vi "From Binary.vi"(8 "error in (no error)":errorcluster, 9 "byte order":T1(ring), 10 "Binary":string, 11 "Double Float in":refnum<class "AbsFunc_One Term_DBL.lvclass">) -> (0 "error out":errorcluster, 2 "Remaning Binary":string, 3 "Double Float out":refnum<class "AbsFunc_One Term_DBL.lvclass">)   [LabVIEW 2021, in "AbsFunc_One Term_DBL.lvclass"]
uses:
  AbsFunc_One Term_DBL.lvclass
  AbsFunc_One Term_DBL.lvclass/AbsFunc_One Term_DBL.ctl
  Abs_Types/Double Float/Abs_Double Float.lvclass
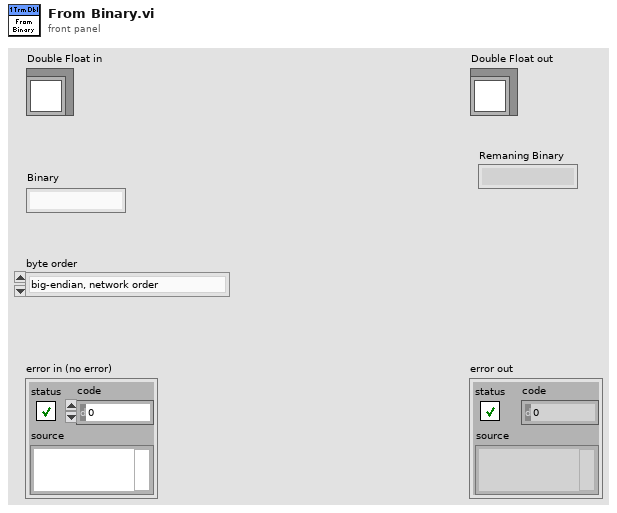
[diagram p1: front panel]
types:
  T1 = enum16{"big-endian, network order", "native, host order", "little-endian"}
  T2 = typedef "One Term_DBL.lvclass/Abstract Type.ctl" = refnum<class "Abs_Double Float.lvclass">
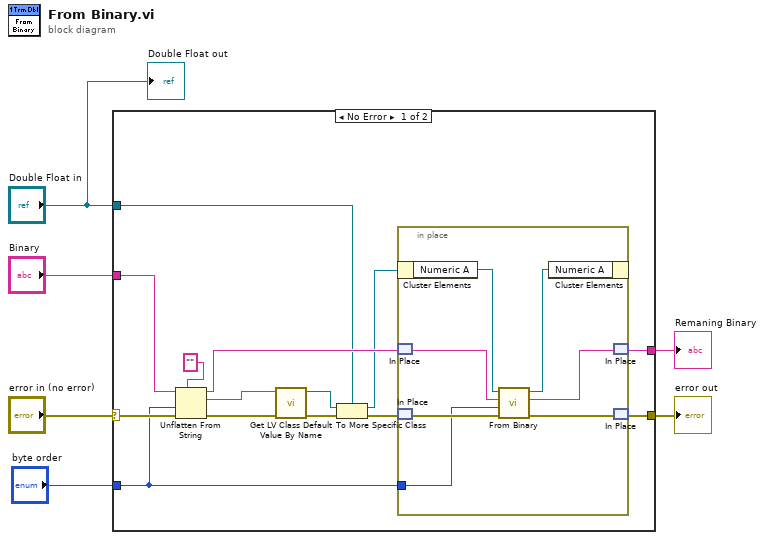
[diagram p0: block diagram]
diagram:
  n1 = case shown="No Error" "error in (no error)" {
    selector: "error in (no error)" -> [w20 w28]
    tunnel: "Binary" -> [w19 w29]
    tunnel: [w12 w28] -> w4
    tunnel: "byte order" -> [w11 _]
    tunnel: [w9 w29] -> w2
    tunnel: "Double Float in" -> [w7 _]
    frame No Error {
      n2 = Unflatten From String(type="", binary string=w19, byte order (0:big-endian, network order)=w11, error in (no error)=w20) -> (rest of the binary string=w10:string, value=w17:string, error out=w16:errorcluster)  [unwired: 1 in]
      n3 = call <vilib>:"Get LV Class Default Value By Name.vi"("error in (no error)"=w16, "class name"=w17) -> ("error out"=w15:errorcluster, "object"=w14:refnum<class>)  [unwired: 8 in]
      n4 = To More Specific Class(target class=w7, reference=w14, error in=w15) -> (specific class reference=w8:refnum<class "AbsFunc_One Term_DBL.lvclass">, error out=w13:errorcluster)
      n5 = in-place {
        in-place-border: w11 -> [w23]
        n6 = in-place-cluster #1(w8) -> ("Numeric A"=w25:T2)
        n7 = in-place-match #2(w10) -> (w22:string)
        n8 = in-place-match #3(w13) -> (w27:errorcluster)
        n9 = call-dynamic "From Binary.vi"("error in (no error)"=w27, "byte order"=w23, "Binary"=w22, "Double Float in"=w25) -> ("error out"=w26:errorcluster, "Remaning Binary"=w21:string, "Double Float out"=w24:T2)  [unwired: 5 in]
        n10 = in-place-cluster #1("Numeric A"=w24) -> ()  [unwired: 1 out]
        n11 = in-place-match #2(w21) -> (w9:string)
        n12 = in-place-match #3(w26) -> (w12:errorcluster)
      }
    }
    frame Error {
    }
  }
  "error out" <- w4
  "Remaning Binary" <- w2
  "Double Float out" <- "Double Float in"
